vi "Configure Alarm Limits.vi"(5 "Maximum Limit (100%)":dbl=100.0 min=0.0 max=100.0 step=1.0 format="%#g", 7 "Minimum Limit (0%)":dbl min=0.0 max=100.0 step=1.0 format="%#g", 8 "error in (no error)":errorcluster, 10 "Node (3)":u8=3 caption="Node" min=3 max=128 step=1, 11 "VISA resource name":refnum<visa-resource-name>) -> (0 "error out":errorcluster, 3 "VISA resource name out":refnum<visa-resource-name>)   [LabVIEW 2024, in "Bronkhorst FLOW-BUS.lvlib"]
doc: "Configures the minimum and maximum values that will cause an alarm if the alarm mode is set to \"Alarm on absolute limits\"."
uses:
  Bronkhorst FLOW-BUS.lvlib
  Private/FLOW-BUS RW.ctl
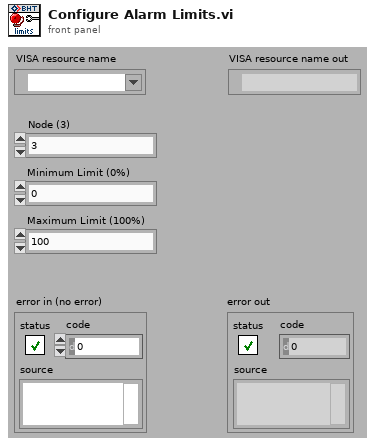
[diagram p1: front panel]
types:
  T1 = typedef "Bronkhorst FLOW-BUS.lvlib/FLOW-BUS RW.ctl" = cluster{"Node Address (3)":u8, "Communication Command":enum16{"Status message", "Send parameter with destination address and 00 response", "Send parameter with destination address", "Request parameter"}, "Process (0)":u16, "Parameter (0)":u16, "Data Type (0: Character)":enum16{"Character", "Integer", "Float or Long", "String"}, "Data for Char, Int, or Long (0)":u32, "Data for Float (0)":sgl, "Data for String":string, "Length of Requested String (0)":u8}
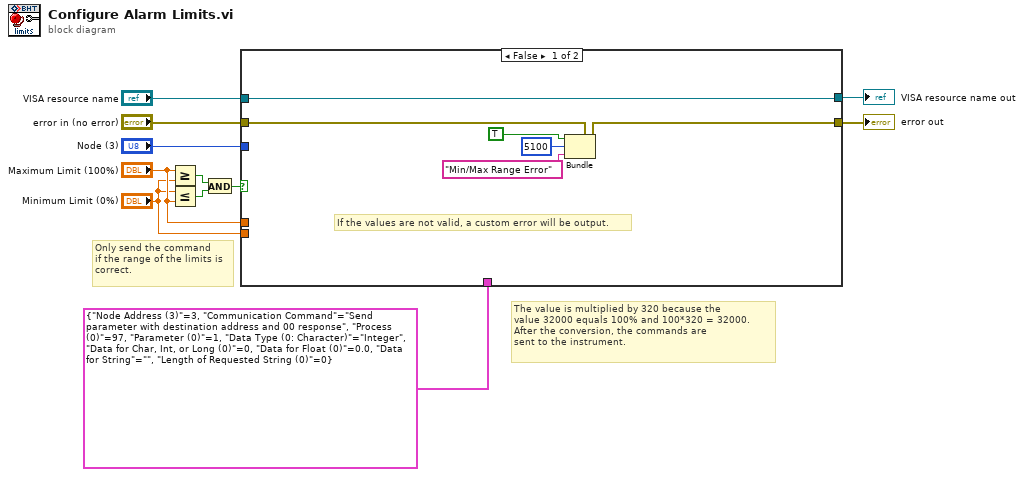
[diagram p0: block diagram]
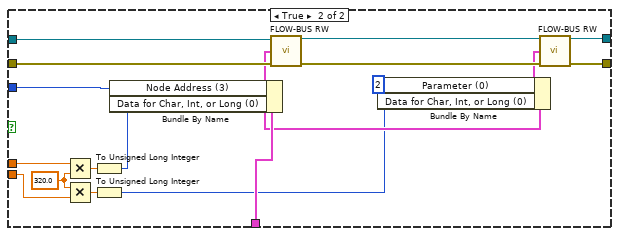
[diagram p2: hidden frame]
diagram:
  # "The value is multiplied by 320 because the \nvalue 32000 equals 100% and 100*320 = 32000.\nAfter the conversion, the commands are \nsent to the instrument."
  # "Only send the command \nif the range of the limits is\ncorrect."
  n1 = Greater Or Equal?(x="Maximum Limit (100%)", y="Minimum Limit (0%)") -> (x >= y?=w10:bool)
  n2 = Less Or Equal?(x="Minimum Limit (0%)", y="Maximum Limit (100%)") -> (x <= y?=w11:bool)
  n3 = And(x=w10, y=w11) -> (x .and. y?=w2:bool)
  n4 = case shown="False" w2 {
    tunnel: "VISA resource name" -> [w17 w30]
    tunnel: "error in (no error)" -> [w16 w27]
    tunnel: [w17 w32] -> w7
    tunnel: [w15 w31] -> w6
    tunnel: "Node (3)" -> [_ w25]
    tunnel: "Maximum Limit (100%)" -> [_ w34]
    tunnel: "Minimum Limit (0%)" -> [_ w33]
    tunnel: T1 {"Node Address (3)"=3, "Communication Command"=enum."Send parameter with destination address and 00 response", "Process (0)"=97, "Parameter (0)"=1, "Data Type (0: Character)"=enum."Integer", "Data for Char, Int, or Long (0)"=0, "Data for Float (0)"=0.0, "Data for String"="", "Length of Requested String (0)"=0} ("FLOW-BUS Command Settings") -> [_ w26]
    frame False {
      # "If the values are not valid, a custom error will be output."
      n5 = Bundle(cluster=w16, "status"=TRUE, "code"=5100, "source"="Min/Max Range Error") -> (w15:errorcluster)
    }
    frame True {
      w35 = 320.0
      n6 = Multiply(x=w34, y=w35) -> (x*y=w21:dbl)
      n7 = Multiply(x=w35, y=w33) -> (x*y=w19:dbl)
      n8 = To Unsigned Long Integer(number=w21) -> (unsigned 32bit integer=w20:u32)
      n9 = To Unsigned Long Integer(number=w19) -> (unsigned 32bit integer=w18:u32)
      n10 = Bundle By Name(cluster=w26, "Node Address (3)"=w25, "Data for Char, Int, or Long (0)"=w20) -> (w23:T1)
      n11 = call "FLOW-BUS RW.vi"("VISA resource name"=w30, "FLOW-BUS Command Settings"=w23, "error in (no error)"=w27) -> ("VISA resource name out"=w29:refnum<visa-resource-name>, "error out"=w28:errorcluster)  [unwired: 8 in, 3 out]
      n12 = Bundle By Name(cluster=w23, "Parameter (0)"=u16 2 ("Parameter"), "Data for Char, Int, or Long (0)"=w18) -> (w24:T1)
      n13 = call "FLOW-BUS RW.vi"("VISA resource name"=w29, "FLOW-BUS Command Settings"=w24, "error in (no error)"=w28) -> ("VISA resource name out"=w32:refnum<visa-resource-name>, "error out"=w31:errorcluster)  [unwired: 8 in, 3 out]
    }
  }
  "VISA resource name out" <- w7
  "error out" <- w6
